vi "CoboltLaser_DriveCurrentSet.vi"(0 "ComPort":refnum<visa-resource-name>, 1 "LaserCurrent (A)":dbl format="%.3g", 3 "CheckResponse":bool=TRUE, 7 "ErrorIn":errorcluster) -> (20 "ComPortOut":refnum<visa-resource-name>, 27 "ErrorOut":errorcluster)   [LabVIEW 2012, in "Cobolt.lvclass"]
doc: "Use this template to build a VI to use as a subVI."
uses:
  Template/Cobolt.lvclass
panel:
  out "ResponseOK":bool
  out "Response":string
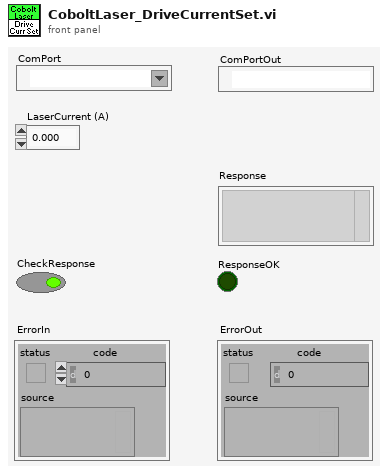
[diagram p1: front panel]
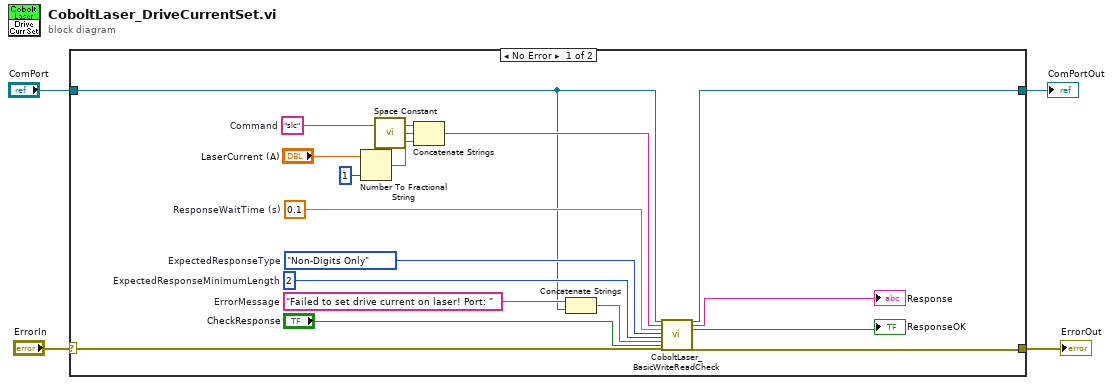
[diagram p0: block diagram]
diagram:
  n1 = case shown="No Error" "ErrorIn" {
    selector: "ErrorIn" -> [w22 w24]
    tunnel: [w21 w24] -> w3
    tunnel: "ComPort" -> [w6 w23]
    tunnel: [w5 w23] -> w1
    frame No Error {
      w18 = 2  # ExpectedResponseMinimumLength
      w19 = enum16{"Any", "Digits Only", "Non-Digits Only"}."Non-Digits Only"  # ExpectedResponseType
      w20 = 0.1  # ResponseWaitTime (s)
      w14 = "Failed to set drive current on laser! Port: "  # ErrorMessage
      w12 = "slc"  # Command
      n2 = Number To Fractional String(number="LaserCurrent (A)", precision (6)=i16 1) -> (F-format string=w9:string)  [unwired: 2 in]
      n3 = call <vilib>:"Space Constant.vi"() -> ("String"=w11:string)
      n4 = Concatenate Strings(w12, w11, w9) -> (w8:string)
      n5 = Concatenate Strings(w14, w6) -> (w13:string)
      n6 = call "CoboltLaser_BasicWriteReadCheck.vi"("ComPort"=w6, "Command"=w8, "ResponseWaitTime (s)"=w20, "ExpectedResponseType"=w19, "ExpectedResponseMinimumLength"=w18, "ErrorMessage"=w13, "CheckResponse"="CheckResponse", "error in (no error)"=w22) -> ("ComPortOut"=w5:refnum<visa-resource-name>, "Response"=→"Response":string, "ResponseOK"=→"ResponseOK":bool, "error out"=w21:errorcluster)  [unwired: 16 in]
    }
    frame Error {
    }
  }
  "ErrorOut" <- w3
  "ComPortOut" <- w1
